vi "Autonomous Independent.vi"() -> ()   [LabVIEW 2014]
doc: "This VI is called when autonomous begins, and will automatically be terminated when autonomous ends. You can carry out timed or sensor driven robot movement independently without needing to return to the caller."
uses:
  <vilib>/Rock Robotics/WPI/Joystick/WPI_JoystickGetSetRefNum.vi
  <vilib>/Rock Robotics/Network Tables/SD Write Numeric Array.vi
  Robot Global Data.vi
  <vilib>/Rock Robotics/WPI/RobotDrive/WPI_RobotDriveMecanumDrive_Cartesian.vi
  <vilib>/Rock Robotics/WPI/RobotDrive/WPI_RobotDriveMecanumDrive_Polar.vi
panel:
  out "Current Movement, for debugging":T1 {"Z Joystick Value" scale=-1.0..1.0; "Y Joystick Value" scale=1.0..-1.0; "X Joystick Value" scale=-1.0..1.0}
  in  "Array of robot movements":T2(array[cluster]) {"Z Joystick Value" scale=-1.0..1.0; "Y Joystick Value" scale=1.0..-1.0; "X Joystick Value" scale=-1.0..1.0}
  # "Be sure to right-click and choose Data Operations>>Make Current Value default if you want to save the array values with the VI"
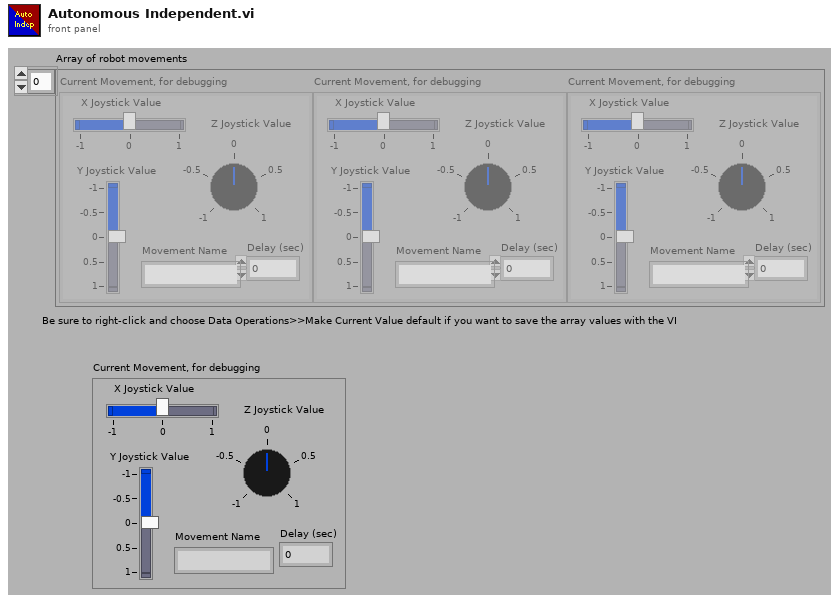
[diagram p1: front panel]
types:
  T1 = cluster{"X Joystick Value":dbl, "Y Joystick Value":dbl, "Z Joystick Value":dbl, "Delay (sec)":dbl, "Movement Name":string}
  T2 = cluster{"X Joystick Value":dbl, "Y Joystick Value":dbl, "Z Joystick Value":dbl, "Delay (sec)":dbl, "Movement Name":string}[]
  T3 = typedef "WPI_SwitchDevRef.ctl" = cluster{"DevStatus":errorcluster, "DIO Channel":T4, "Controller":T5, "CntIndex":T6, "Normally Closed":bool}
  T4 = typedef "FPGA_DIOChannel.ctl" = enum8{"DIO 0", "DIO 1", "DIO 2", "DIO 3", "DIO 4", "DIO 5", "DIO 6", "DIO 7", "DIO 8", "DIO 9", "DIO MXP 0", "DIO MXP 1", "DIO MXP 2", "DIO MXP 3", "DIO MXP 4", "DIO MXP 5", "DIO MXP 6", "DIO MXP 7", "DIO MXP 8", "DIO MXP 9", "DIO MXP 10", "DIO MXP 11", "DIO MXP 12", "DIO MXP 13", "DIO MXP 14", "DIO MXP 15", "Invalid"}
  T5 = typedef "FPGA_TypedefDigitalModule.ctl" = enum16{"Controller 1"}
  T6 = typedef "FPGA_CounterCtrSystemIndex.ctl" = enum8{"Ctr 0", "Ctr 1", "Ctr 2", "Ctr 3", "Ctr 4", "Ctr 5", "Ctr 6", "Ctr 7", "Invalid"}
  T7 = typedef "WPI_RobotDriveDevRef.ctl" = cluster{"DevStatus":errorcluster, "Motors[]":T8[], "Square Inputs":bool, "Max Output":dbl}
  T8 = typedef "WPI_MotorControlDeviceRef.ctl" = cluster{"DeviceStatus":errorcluster, "Type":T9, "PWM":cluster{"Controller":T5, "PWM Channel":T10, "DeadBand":T11}, "CAN":cluster{"Device Number":u8, "Control Mode":T12, "Semaphore":T13, "Max Vout":dbl, "TalonSRX Control Mode":T14}, "Invert":bool, "TransformRef":T15, "InvTransformRef":T15}
  T9 = typedef "WPI_MotorControlType.ctl" = enum16{"PWM", "CAN", "CANTalonSRX"}
  T10 = typedef "FPGA_DIOPWMChannel.ctl" = enum8{"PWM 0", "PWM 1", "PWM 2", "PWM 3", "PWM 4", "PWM 5", "PWM 6", "PWM 7", "PWM 8", "PWM 9", "PWM MXP 0", "PWM MXP 1", "PWM MXP 2", "PWM MXP 3", "PWM MXP 4", "PWM MXP 5", "PWM MXP 6", "PWM MXP 7", "PWM MXP 8", "PWM MXP 9", "Invalid"}
  T11 = typedef "WPI_PWMDeadband.ctl" = cluster{"Name":string, "maxPositivePwm":i32, "minPositivePwm":i32, "centerPwm":i32, "maxNegativePwm":i32, "minNegativePwm":i32, "angularRange":u16}
  T12 = typedef "WPI_CANJaguar_ControlMode.ctl" = enum8{"Percent VBus", "Current", "Speed", "Position", "Voltage"}
  T13 = typedef "Semaphore RefNum" = refnum<k1>
  T14 = typedef "WPI_CANTalonSRX_APIControlMode.ctl" = enum8{"Percent VBus", "Speed", "Position", "Slave", "Unchanged / Invalid"}
  T15 = typedef "WPI_PWMTransform_ConPane.ctl" = refnum<vi>
  T16 = cluster{"Distance (ft)":dbl, "Center":cluster{dbl, dbl}, "Normalized Rect":cluster{"Numeric":dbl, "Numeric 2":dbl, "Numeric 3":dbl, "Numeric 5":dbl}}[]
  T17 = cluster{"Distance (ft)":dbl, "Center":cluster{dbl, dbl}, "Normalized Rect":cluster{"Numeric":dbl, "Numeric 2":dbl, "Numeric 3":dbl, "Numeric 5":dbl}}
  T18 = typedef "WPI_JoystickDevRef.ctl" = cluster{"Device":T19}
  T19 = typedef "WPI_JoystickDeviceEnum.ctl" = enum16{"USB 0", "USB 1", "USB 2", "USB 3", "USB 4", "USB 5"}
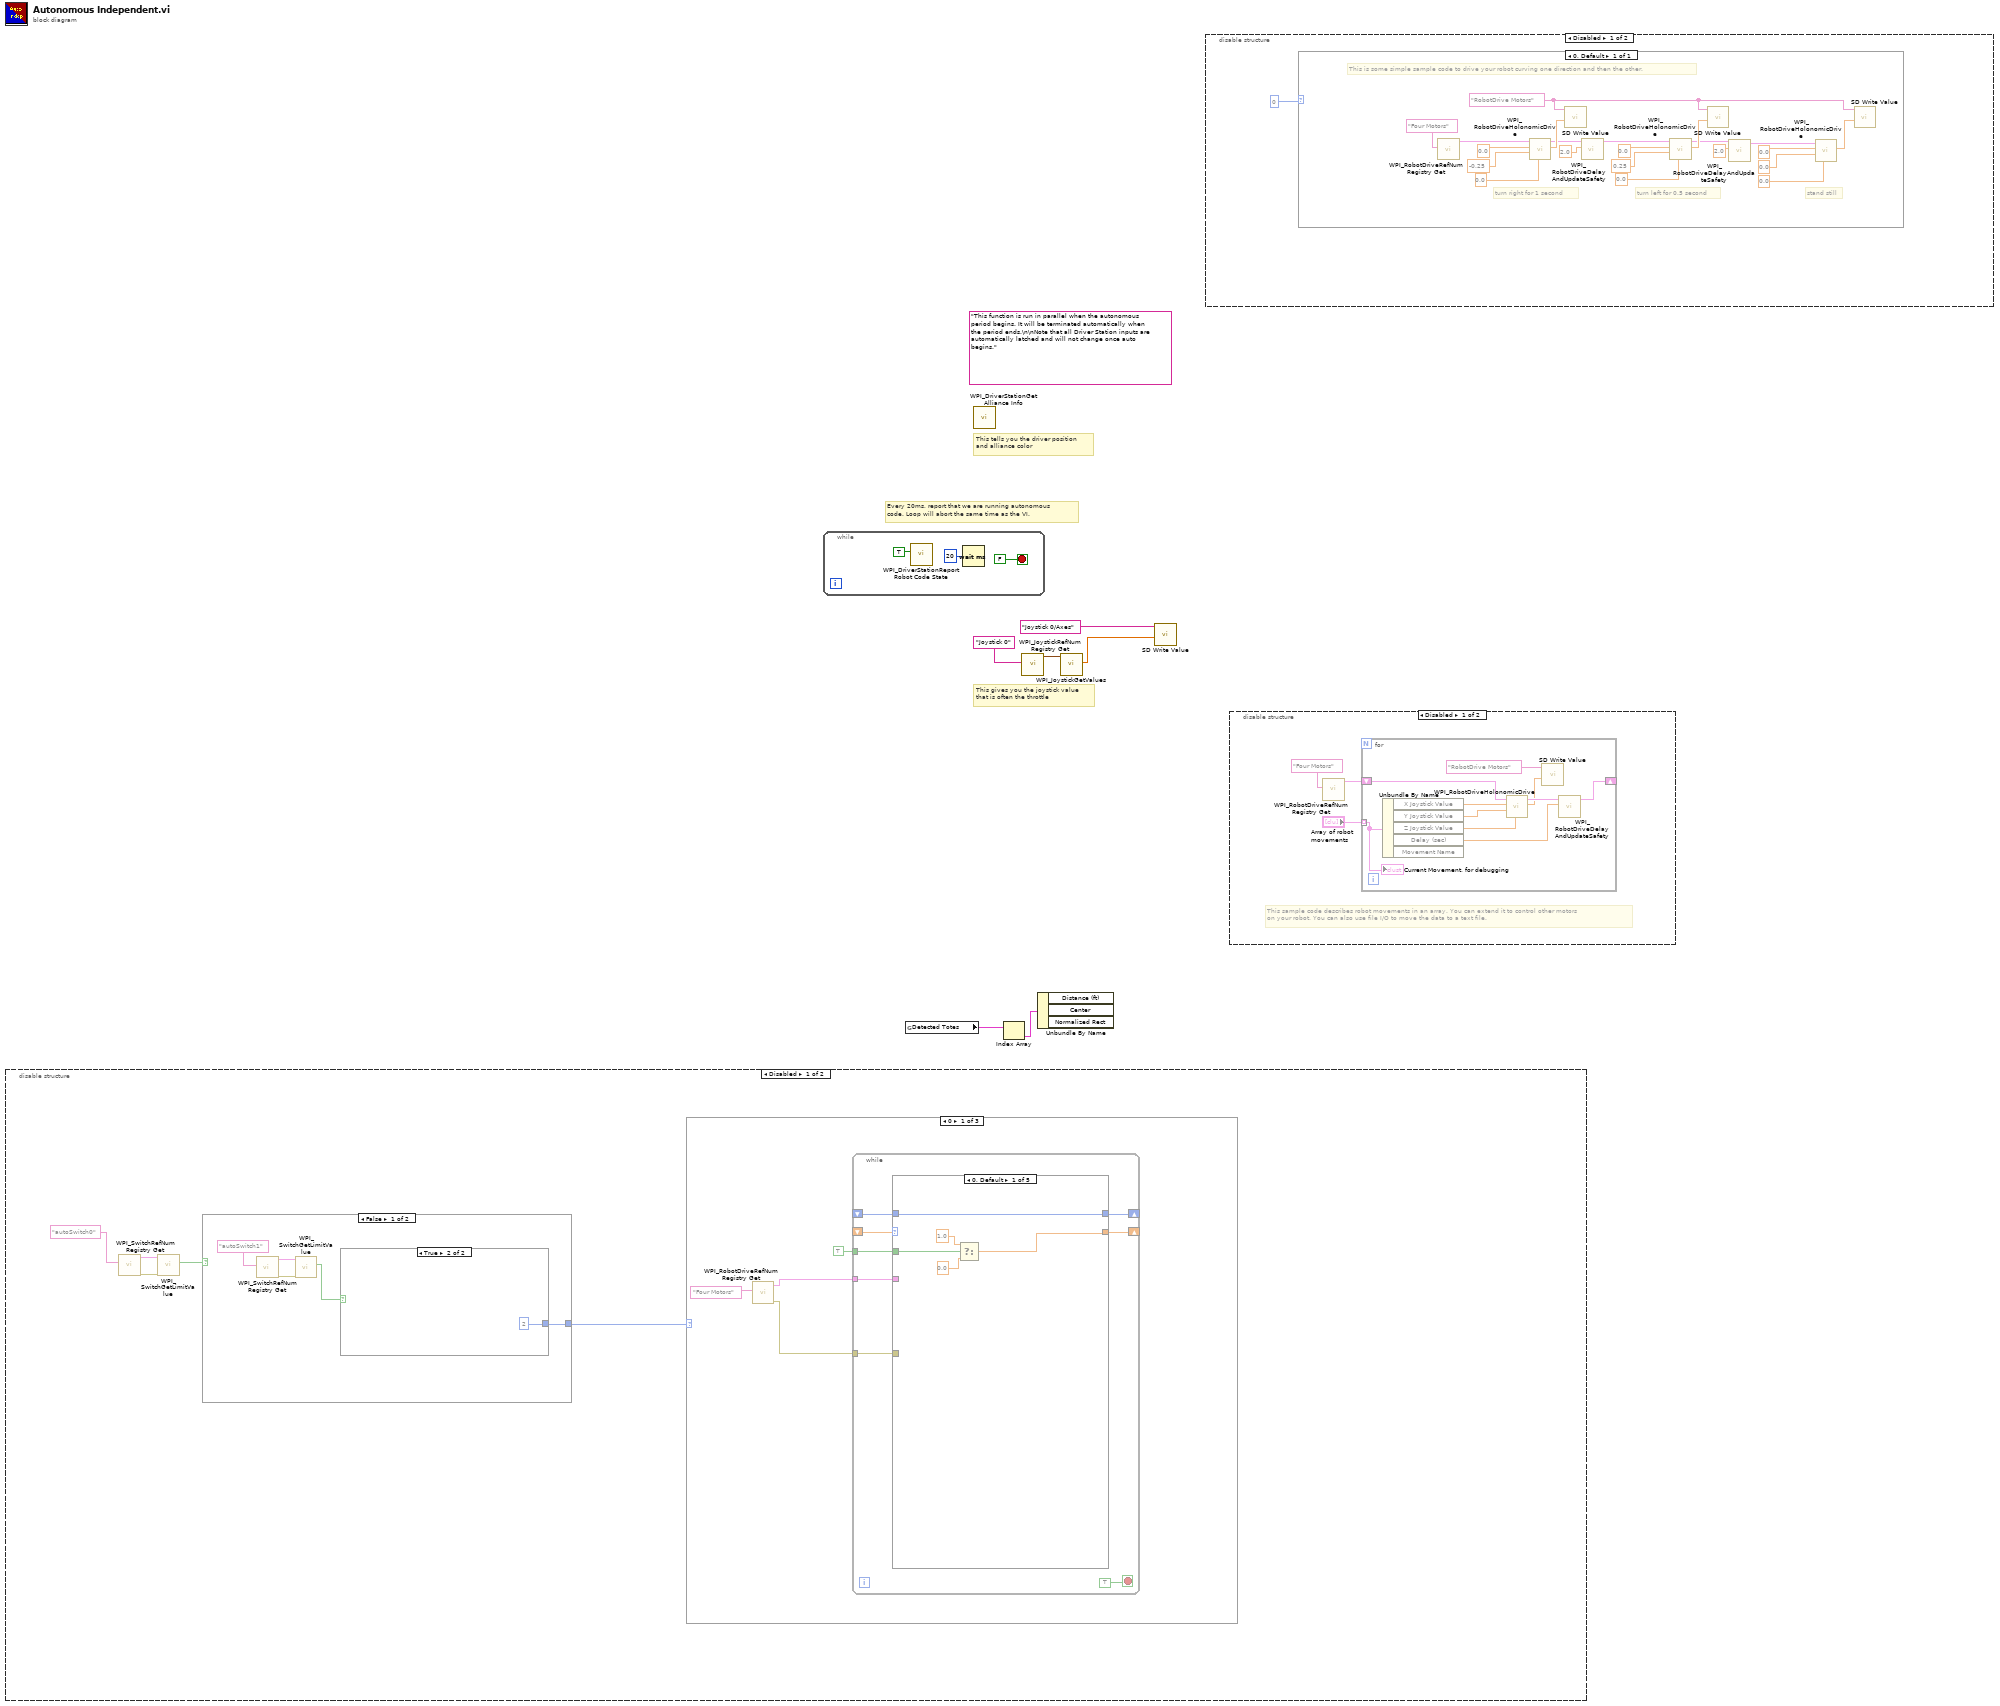
[diagram p0: block diagram]
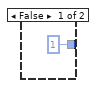
[diagram p2: hidden frame]
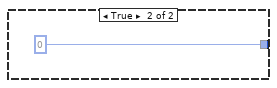
[diagram p3: hidden frame]
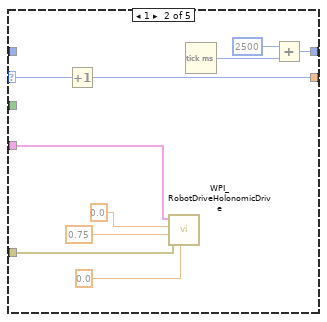
[diagram p4: hidden frame]
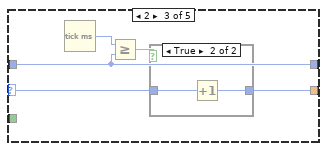
[diagram p5: hidden frame]
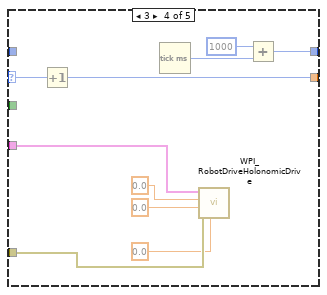
[diagram p7: hidden frame]
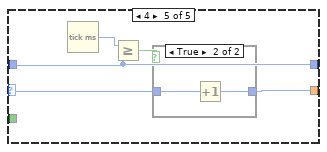
[diagram p8: hidden frame]
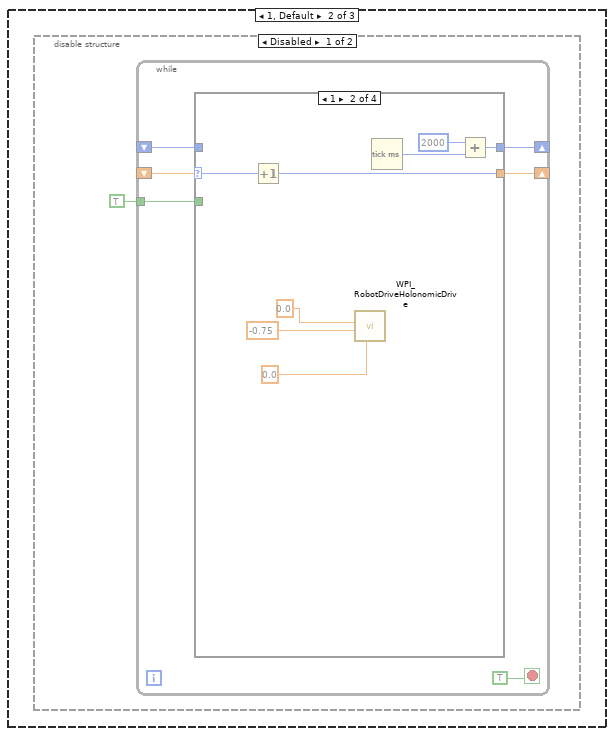
[diagram p10: hidden frame]
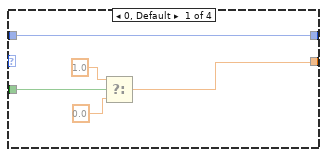
[diagram p11: hidden frame]
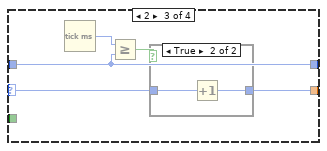
[diagram p12: hidden frame]
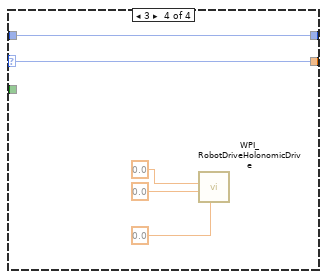
[diagram p14: hidden frame]
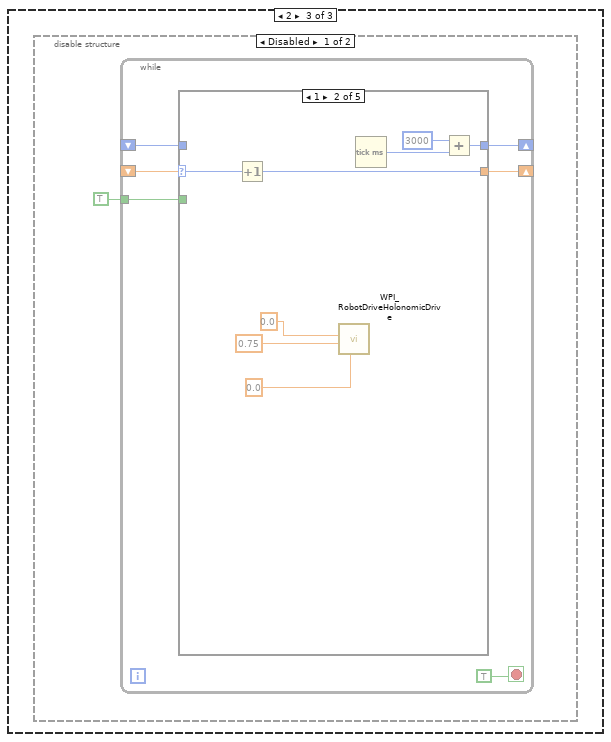
[diagram p16: hidden frame]
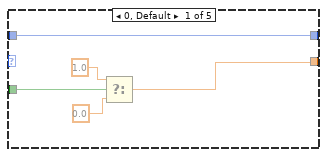
[diagram p17: hidden frame]
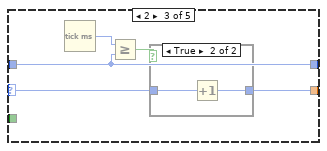
[diagram p18: hidden frame]
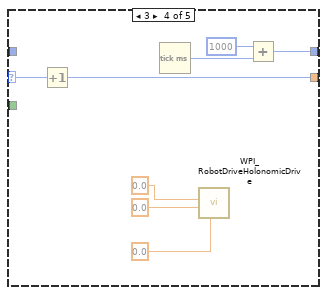
[diagram p20: hidden frame]
diagram:
  (unwired) "This function is run in parallel when the autonomous period begins. It will be terminated automatically when the period ends.\n\nNote that all Driver Station inputs are automatically latched and will not change once auto begins."
  # "Every 20ms, report that we are running autonomous\ncode. Loop will abort the same time as the VI."
  # "This gives you the joystick value\nthat is often the throttle"
  # "This tells you the driver position\nand alliance color"
  n1 = disable-structure shown="Disabled" {
    frame Disabled {
      n2 = call <vilib>:"WPI_SwitchRefNum Registry Get.vi"("refnum name"="autoSwitch0") -> ("error out"=w10:errorcluster, "SwitchDevRef"=w11:T3)  [unwired: 9 in]
      n3 = call <vilib>:"WPI_SwitchGetLimitValue.vi"("error in (no error)"=w10, "SwitchDevRef"=w11) -> ("Switch Pressed"=w9:bool)  [unwired: 7 in, 2 out]
      n4 = case shown="False" w9 {
        tunnel: [w12 0] -> w7
        frame False {
          n5 = call <vilib>:"WPI_SwitchRefNum Registry Get.vi"("refnum name"="autoSwitch1") -> ("error out"=w16:errorcluster, "SwitchDevRef"=w15:T3)  [unwired: 9 in]
          n6 = call <vilib>:"WPI_SwitchGetLimitValue.vi"("error in (no error)"=w16, "SwitchDevRef"=w15) -> ("Switch Pressed"=w13:bool)  [unwired: 7 in, 2 out]
          n7 = case shown="True" w13 {
            tunnel: [1 2] -> w12
            frame False {
            }
            frame True {
            }
          }
        }
        frame True {
        }
      }
      n8 = case shown="0" w7 {
        frame 0 {
          n9 = call <vilib>:"WPI_RobotDriveRefNum Registry Get.vi"("refnum name"="Four Motors") -> ("error out"=w20:errorcluster, "RobotDriveDevRef"=w21:T7)  [unwired: 1 in, 8 out]
          n10 = while {
            shift-right: [w30] -> _
            shift-left: _ -> [w29]
            shift-right: [w28] -> _
            shift-left: _ -> [w27]
            tunnel: TRUE ("Switch Pressed") -> [w26]
            tunnel: w21 -> [w25]
            tunnel: w20 -> [w24]
            stop <- TRUE stop-if-true
            n11 = case shown="0, Default" w29 {
              selector: w29 -> [_ w46 w50 w63 w67]
              tunnel: [w34 w45 w49 w62 w66] -> w30
              tunnel: [w33 w44 w47 w61 w65] -> w28
              tunnel: w27 -> [w33 _ w47 _ w65]
              tunnel: w26 -> [w32 _ _ _ _]
              tunnel: w25 -> [_ w41 _ w59 _]
              tunnel: w24 -> [_ w40 _ w58 _]
              frame 0, Default {
                n12 = Select(t=1.0, s=w32, f=0.0) -> (s? t:f=w34:dbl)
              }
              frame 1 {
                n13 = Increment(x=w46) -> (x+1=w45:i32)
                n14 = call-poly <vilib>:"WPI_RobotDriveHolonomicDrive.vi"("Rotation"=0.0, "error in (no error)"=w40, "Y"=0.75, "X"=0.0, "RobotDriveDevRef"=w41) -> ()  [unwired: 4 in, 3 out]
                n15 = Tick Count (ms)() -> (millisecond timer value=w43:u32)
                n16 = Add(x=u32 2500, y=w43) -> (x+y=w44:u32)
              }
              frame 2 {
                n17 = Tick Count (ms)() -> (millisecond timer value=w48:u32)
                n18 = Greater Or Equal?(x=w48, y=w47) -> (x >= y?=w51:bool)
                n19 = case shown="True" w51 {
                  tunnel: [w52 w53] -> w49
                  tunnel: w50 -> [w52 w54]
                  frame False {
                  }
                  frame True {
                    n20 = Increment(x=w54) -> (x+1=w53:i32)
                  }
                }
              }
              frame 3 {
                n21 = Increment(x=w63) -> (x+1=w62:i32)
                n22 = Tick Count (ms)() -> (millisecond timer value=w64:u32)
                n23 = call-poly <vilib>:"WPI_RobotDriveHolonomicDrive.vi"("Rotation"=0.0, "error in (no error)"=w58, "Direction"=0.0, "Magnitude"=0.0, "RobotDriveDevRef"=w59) -> ()  [unwired: 4 in, 3 out]
                n24 = Add(x=u32 1000, y=w64) -> (x+y=w61:u32)
              }
              frame 4 {
                n25 = Tick Count (ms)() -> (millisecond timer value=w68:u32)
                n26 = Greater Or Equal?(x=w68, y=w65) -> (x >= y?=w69:bool)
                n27 = case shown="True" w69 {
                  tunnel: [w70 w71] -> w66
                  tunnel: w67 -> [w70 w72]
                  frame False {
                  }
                  frame True {
                    n28 = Increment(x=w72) -> (x+1=w71:i32)
                  }
                }
              }
            }
          }
        }
        frame 1, Default {
          n29 = disable-structure shown="Disabled" {
            frame Disabled {
              n30 = while {
                shift-right: [w78] -> _
                shift-left: _ -> [w77]
                shift-right: [w76] -> _
                shift-left: _ -> [w75]
                tunnel: TRUE ("Switch Pressed") -> [w74]
                stop <- TRUE stop-if-true
                n31 = case shown="1" w77 {
                  selector: w77 -> [_ w92 w96 w102]
                  tunnel: [w82 w91 w95 w102] -> w78
                  tunnel: [w81 w90 w93 w101] -> w76
                  tunnel: w75 -> [w81 _ w93 w101]
                  tunnel: w74 -> [w80 _ _ _]
                  frame 0, Default {
                    n32 = Select(t=1.0, s=w80, f=0.0) -> (s? t:f=w82:dbl)
                  }
                  frame 1 {
                    n33 = Increment(x=w92) -> (x+1=w91:i32)
                    n34 = call-poly <vilib>:"WPI_RobotDriveHolonomicDrive.vi"("Rotation"=0.0, "Y"=-0.75, "X"=0.0) -> ()  [unwired: 6 in, 3 out]
                    n35 = Tick Count (ms)() -> (millisecond timer value=w89:u32)
                    n36 = Add(x=u32 2000, y=w89) -> (x+y=w90:u32)
                  }
                  frame 2 {
                    n37 = Tick Count (ms)() -> (millisecond timer value=w94:u32)
                    n38 = Greater Or Equal?(x=w94, y=w93) -> (x >= y?=w97:bool)
                    n39 = case shown="True" w97 {
                      tunnel: [w98 w99] -> w95
                      tunnel: w96 -> [w98 w100]
                      frame False {
                      }
                      frame True {
                        n40 = Increment(x=w100) -> (x+1=w99:i32)
                      }
                    }
                  }
                  frame 3 {
                    n41 = call-poly <vilib>:"WPI_RobotDriveHolonomicDrive.vi"("Rotation"=0.0, "Direction"=0.0, "Magnitude"=0.0) -> ()  [unwired: 6 in, 3 out]
                  }
                }
              }
            }
            frame Enabled {
            }
          }
        }
        frame 2 {
          n42 = disable-structure shown="Disabled" {
            frame Disabled {
              n43 = while {
                shift-right: [w111] -> _
                shift-left: _ -> [w110]
                shift-right: [w109] -> _
                shift-left: _ -> [w108]
                tunnel: TRUE ("Switch Pressed") -> [w107]
                stop <- TRUE stop-if-true
                n44 = case shown="1" w110 {
                  selector: w110 -> [_ w125 w129 w140 w144]
                  tunnel: [w115 w124 w128 w139 w143] -> w111
                  tunnel: [w114 w123 w126 w138 w142] -> w109
                  tunnel: w108 -> [w114 _ w126 _ w142]
                  tunnel: w107 -> [w113 _ _ _ _]
                  frame 0, Default {
                    n45 = Select(t=1.0, s=w113, f=0.0) -> (s? t:f=w115:dbl)
                  }
                  frame 1 {
                    n46 = Increment(x=w125) -> (x+1=w124:i32)
                    n47 = call-poly <vilib>:"WPI_RobotDriveHolonomicDrive.vi"("Rotation"=0.0, "Y"=0.75, "X"=0.0) -> ()  [unwired: 6 in, 3 out]
                    n48 = Tick Count (ms)() -> (millisecond timer value=w122:u32)
                    n49 = Add(x=u32 3000, y=w122) -> (x+y=w123:u32)
                  }
                  frame 2 {
                    n50 = Tick Count (ms)() -> (millisecond timer value=w127:u32)
                    n51 = Greater Or Equal?(x=w127, y=w126) -> (x >= y?=w130:bool)
                    n52 = case shown="True" w130 {
                      tunnel: [w131 w132] -> w128
                      tunnel: w129 -> [w131 w133]
                      frame False {
                      }
                      frame True {
                        n53 = Increment(x=w133) -> (x+1=w132:i32)
                      }
                    }
                  }
                  frame 3 {
                    n54 = Increment(x=w140) -> (x+1=w139:i32)
                    n55 = Tick Count (ms)() -> (millisecond timer value=w141:u32)
                    n56 = call-poly <vilib>:"WPI_RobotDriveHolonomicDrive.vi"("Rotation"=0.0, "Direction"=0.0, "Magnitude"=0.0) -> ()  [unwired: 6 in, 3 out]
                    n57 = Add(x=u32 1000, y=w141) -> (x+y=w138:u32)
                  }
                  frame 4 {
                    n58 = Tick Count (ms)() -> (millisecond timer value=w145:u32)
                    n59 = Greater Or Equal?(x=w145, y=w142) -> (x >= y?=w146:bool)
                    n60 = case shown="True" w146 {
                      tunnel: [w147 w148] -> w143
                      tunnel: w144 -> [w147 w149]
                      frame False {
                      }
                      frame True {
                        n61 = Increment(x=w149) -> (x+1=w148:i32)
                      }
                    }
                  }
                }
              }
            }
            frame Enabled {
            }
          }
        }
      }
    }
    frame Enabled {
    }
  }
  n62 = while {
    stop <- FALSE stop-if-true
    n63 = call <vilib>:"WPI_DriverStationReport Robot Code State.vi"("Autonomous"=TRUE) -> ()  [unwired: 10 in, 1 out]
    n64 = Wait (ms)(milliseconds to wait=u32 20) -> ()  [unwired: 1 out]
  }
  n65 = global read "Robot Global Data.vi" "Detected Totes"() -> (w2:T16)
  n66 = call <vilib>:"WPI_DriverStationGet Alliance Info.vi"() -> ()  [unwired: 12 out]
  n67 = Index Array(array=w2) -> (element=w1:T17)  [unwired: 1 in]
  n68 = call <vilib>:"WPI_JoystickRefNum Registry Get.vi"("refnum name"="Joystick 0") -> ("JoystickDevRef"=w5:T18)  [unwired: 1 in, 9 out]
  n69 = Unbundle By Name(w1) -> ()  [unwired: 3 out]
  n70 = call <vilib>:"WPI_JoystickGetValues.vi"("JoystickDevRef"=w5) -> ("Axes"=w3:dbl[])  [unwired: 6 in, 4 out]
  n71 = call-poly <vilib>:"SD Write Value.vi"("Numeric Array"=w3, "Name"="Joystick 0/Axes") -> ()  [unwired: 8 in, 2 out]
  n72 = disable-structure shown="Disabled" {
    frame Disabled {
      n73 = case shown="0, Default" 0 {
        frame 0, Default {
          w168 = "RobotDrive Motors" ("Name")
          # "This is some simple sample code to drive your robot curving one direction and then the other."
          # "stand still"
          # "turn left for 0.5 second"
          # "turn right for 1 second"
          n74 = call <vilib>:"WPI_RobotDriveRefNum Registry Get.vi"("refnum name"="Four Motors") -> ("RobotDriveDevRef"=w167:T7)  [unwired: 1 in, 9 out]
          n75 = call-poly <vilib>:"WPI_RobotDriveHolonomicDrive.vi"("Rotation"=0.0, "Y"=-0.25 ("X axis value"), "X"=0.0 ("X axis value"), "RobotDriveDevRef"=w167) -> ("Motor Values"=w172:dbl[], "RobotDriveDevRef"=w160:T7)  [unwired: 5 in, 1 out]
          n76 = call-poly <vilib>:"SD Write Value.vi"("Numeric Array"=w172, "Name"=w168) -> ()  [unwired: 8 in, 2 out]
          n77 = call <vilib>:"WPI_RobotDriveDelayAndUpdateSafety.vi"("Delay (s)"=2.0, "RobotDriveDevRef"=w160) -> ("RobotDriveDevRef 2"=w161:T7)  [unwired: 8 in, 1 out]
          n78 = call-poly <vilib>:"WPI_RobotDriveHolonomicDrive.vi"("Rotation"=0.0, "Y"=0.25 ("X axis value"), "X"=0.0 ("X axis value"), "RobotDriveDevRef"=w161) -> ("Motor Values"=w173:dbl[], "RobotDriveDevRef"=w162:T7)  [unwired: 5 in, 1 out]
          n79 = call-poly <vilib>:"SD Write Value.vi"("Numeric Array"=w173, "Name"=w168) -> ()  [unwired: 8 in, 2 out]
          n80 = call <vilib>:"WPI_RobotDriveDelayAndUpdateSafety.vi"("Delay (s)"=2.0, "RobotDriveDevRef"=w162) -> ("RobotDriveDevRef 2"=w163:T7)  [unwired: 8 in, 1 out]
          n81 = call-poly <vilib>:"WPI_RobotDriveHolonomicDrive.vi"("Rotation"=0.0 ("X axis value"), "Y"=0.0 ("X axis value"), "X"=0.0 ("X axis value"), "RobotDriveDevRef"=w163) -> ("Motor Values"=w174:dbl[])  [unwired: 5 in, 2 out]
          n82 = call-poly <vilib>:"SD Write Value.vi"("Numeric Array"=w174, "Name"=w168) -> ()  [unwired: 8 in, 2 out]
        }
      }
    }
    frame Enabled {
    }
  }
  n83 = disable-structure shown="Disabled" {
    frame Disabled {
      # "This sample code describes robot movements in an array. You can extend it to control other motors\non your robot. You can also use file I/O to move the data to a text file."
      n84 = call <vilib>:"WPI_RobotDriveRefNum Registry Get.vi"("refnum name"="Four Motors") -> ("RobotDriveDevRef"=w176:T7)  [unwired: 1 in, 9 out]
      n85 = for {
        shift-right: [w184] -> _
        shift-left: w176 -> [w185]
        tunnel: "Array of robot movements" -> [w180] mode=indexing
        n86 = Unbundle By Name(w180) -> ("X Joystick Value"=w183:dbl, "Y Joystick Value"=w182:dbl, "Z Joystick Value"=w179:dbl, "Delay (sec)"=w181:dbl)  [unwired: 1 out]
        n87 = call-poly <vilib>:"WPI_RobotDriveHolonomicDrive.vi"("Rotation"=w179, "Y"=w182, "X"=w183, "RobotDriveDevRef"=w185) -> ("Motor Values"=w178:dbl[], "RobotDriveDevRef"=w186:T7)  [unwired: 5 in, 1 out]
        n88 = call-poly <vilib>:"SD Write Value.vi"("Numeric Array"=w178, "Name"="RobotDrive Motors") -> ()  [unwired: 8 in, 2 out]
        n89 = call <vilib>:"WPI_RobotDriveDelayAndUpdateSafety.vi"("Delay (s)"=w181, "RobotDriveDevRef"=w186) -> ("RobotDriveDevRef 2"=w184:T7)  [unwired: 8 in, 1 out]
        "Current Movement, for debugging" <- w180
      }
    }
    frame Enabled {
    }
  }
